vi "Read_DriveOutput.vi"(8 "error in (no error)":errorcluster, 11 "DriveData in":refnum<class "DriveData.lvclass">) -> (0 "error out":errorcluster, 2 "DriveOutput":T1 {"Control Mode" items=["PercentOutput"=0, "Position"=1, "Velocity"=2, "Current"=3, "Follower"=5, "MotionProfile"=6, "MotionMagic"=7, "MotionMagicArc"=8, "MotionProfileArc"=10, "Disabled"=15]}, 3 "DriveData out":refnum<class "DriveData.lvclass">)   [LabVIEW 2017, in "DriveData.lvclass"]
uses:
  DriveData.lvclass
  DriveOutput.ctl
  <vilib>/Rock Robotics/WPI/ThirdParty/Phoenix-LabVIEW/Motor Controller/Controls/CTRE_Phoenix_MotorControl_ControlMode.ctl
  DriveData.lvclass/DriveData.ctl
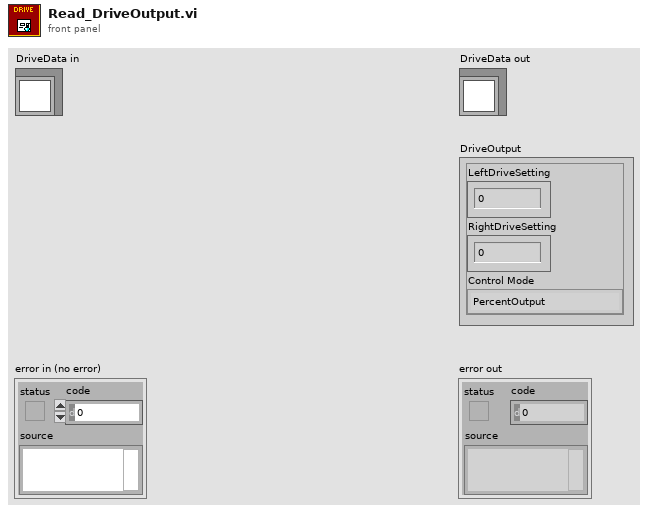
[diagram p1: front panel]
types:
  T1 = typedef "DriveData.lvclass/DriveOutput.ctl" = cluster{"LeftDriveSetting":dbl, "RightDriveSetting":dbl, "Control Mode":T2}
  T2 = typedef "CTRE_Phoenix_MotorControl_ControlMode.ctl" = u16
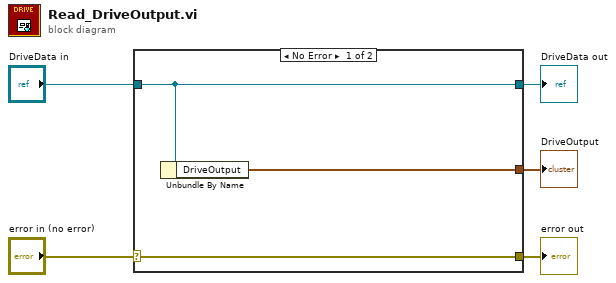
[diagram p0: block diagram]
diagram:
  n1 = case shown="No Error" "error in (no error)" {
    selector: "error in (no error)" -> [w8 w9]
    tunnel: [w8 w9] -> w4
    tunnel: [w7 w10] -> w2
    tunnel: "DriveData in" -> [w7 w10]
    tunnel: [w6 _] -> w1
    frame No Error {
      n2 = Unbundle By Name(w7) -> ("DriveOutput"=w6:T1)
    }
    frame Error {
    }
  }
  "error out" <- w4
  "DriveData out" <- w2
  "DriveOutput" <- w1
